vi "excel显示二维数组.vi"(8 "error in (no error)":errorcluster caption="错误输入（无错误）", 11 "数据二维":string[][](array[string])) -> (0 "error out":errorcluster caption="错误输出")   [LabVIEW 2014]
doc: "该模板用于创建子VI。"
panel:
  out "连接的字符串":string
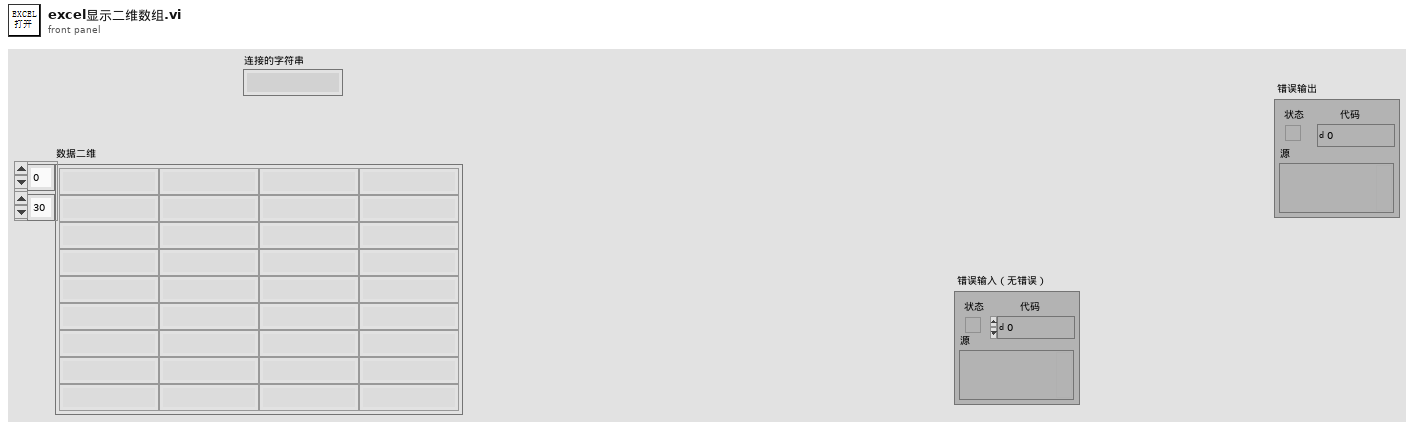
[diagram p1: front panel]
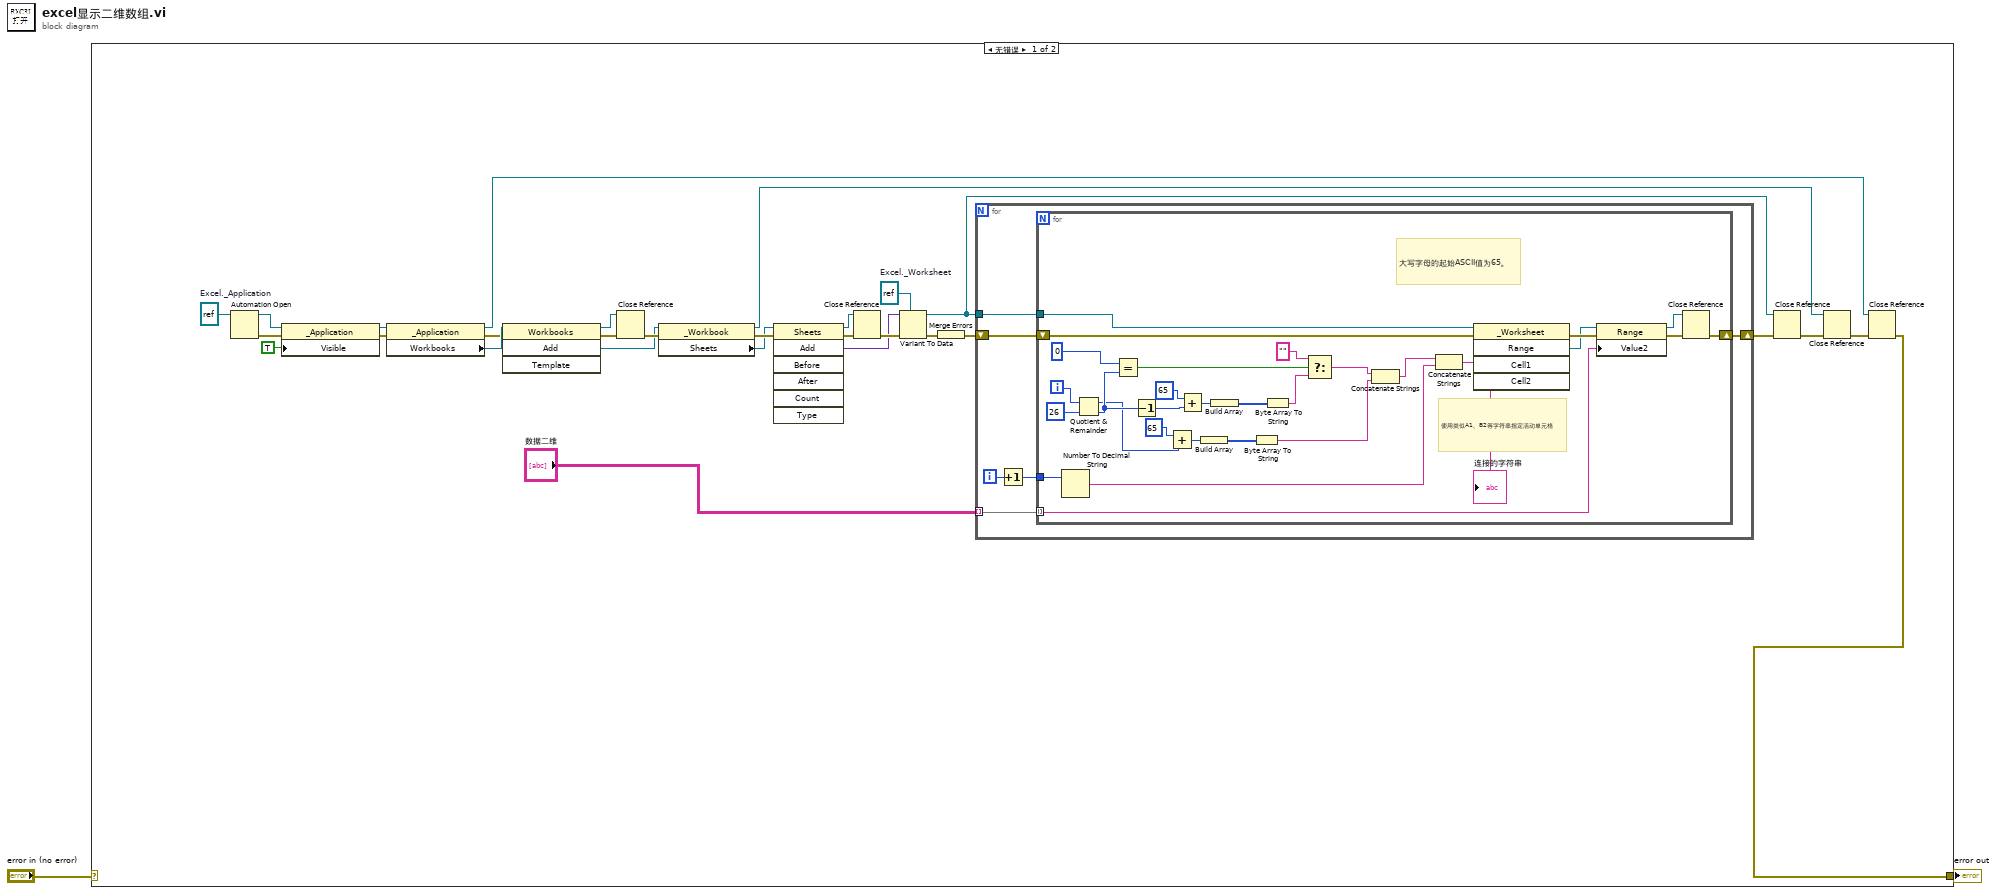
[diagram p0: block diagram]
diagram:
  n1 = case shown="无错误" "error in (no error)" {
    selector: "error in (no error)" -> [_ w67]
    tunnel: [w3 w67] -> w1
    frame No Error {
      w10 = refnum<k7> refnum  # Excel._Worksheet
      w26 = refnum<k7> refnum  # Excel._Application
      n2 = Automation Open(Automation Refnum=w26) -> (Automation Refnum=w27:refnum<k7>, error out=w28:errorcluster)  [unwired: 1 in, 2 out]
      n3 = property class="_Application"(reference=w27, error in=w28, "Visible"=TRUE) -> (reference out=w19:refnum<k7>, error out=w21:errorcluster)
      n4 = property class="_Application"(reference=w19, error in=w21) -> (reference out=w16:refnum<k7>, error out=w24:errorcluster, "Workbooks"=w25:refnum<k7>)
      n5 = invoke class="Workbooks" method="Add"(reference=w25, error in=w24) -> (reference out=w22:refnum<k7>, error out=w23:errorcluster, "Add"=w17:refnum<k7>)  [unwired: 2 in, 1 out]
      n6 = Close Reference(reference=w22, error in (no error)=w23) -> (error out=w18:errorcluster)
      n7 = property class="_Workbook"(reference=w17, error in=w18) -> (reference out=w14:refnum<k7>, error out=w8:errorcluster, "Sheets"=w7:refnum<k7>)
      n8 = invoke class="Sheets" method="Add"(reference=w7, error in=w8) -> (reference out=w11:refnum<k7>, error out=w12:errorcluster, "Add"=w9:variant)  [unwired: 5 in, 4 out]
      n9 = Close Reference(reference=w11, error in (no error)=w12) -> (error out=w13:errorcluster)
      n10 = Variant To Data(error in=w13, type=w10, Variant=w9) -> (data=w15:refnum<k7>, error out=w6:errorcluster)
      n11 = Merge Errors(w6) -> (w5:errorcluster)
      n12 = for {
        shift-right: [w36] -> w29
        shift-left: w5 -> [w37]
        tunnel: w15 -> [w35]
        tunnel: "数据二维" -> [w32] mode=indexing
        i -> [w34]
        n13 = Increment(x=w34) -> (x+1=w33:i32)
        n14 = for {
          shift-right: [w62] -> w36
          shift-left: w37 -> [w60]
          tunnel: w35 -> [w59]
          tunnel: w33 -> [w56]
          tunnel: w32 -> [w64] mode=indexing
          i -> [w53]
          # "使用类似A1、B2等字符串指定活动单元格"
          # "大写字母的起始ASCII值为65。"
          n15 = Number To Decimal String(number=w56) -> (decimal integer string=w55:string)  [unwired: 1 in]
          n16 = Quotient & Remainder(x=w53, y=26) -> (x-y*floor(x/y)=w39:i32, floor(x/y)=w40:i32)
          n17 = Equal?(x=0, y=w40) -> (x = y?=w46:bool)
          n18 = Decrement(x=w40) -> (x-1=w47:i32)
          n19 = Add(x=65, y=w39) -> (x+y=w57:i32)
          n20 = Add(x=65, y=w47) -> (x+y=w49:i32)
          n21 = Build Array(w57) -> (w38:i32[])
          n22 = Build Array(w49) -> (w50:i32[])
          n23 = Byte Array To String(unsigned byte array=w38) -> (string=w42:string)
          n24 = Byte Array To String(unsigned byte array=w50) -> (string=w44:string)
          n25 = Select(t="" ("十进制整型字符串"), s=w46, f=w44) -> (s? t:f=w43:string)
          n26 = Concatenate Strings(w43, w42) -> (w41:string)
          n27 = Concatenate Strings(w41, w55) -> (w54:string)
          "连接的字符串" <- w54
          n28 = invoke class="_Worksheet" method="Range"(reference=w59, error in=w60, "Cell1"=w54) -> (error out=w66:errorcluster, "Range"=w65:refnum<k7>)  [unwired: 2 in, 3 out]
          n29 = property class="Range"(reference=w65, error in=w66, "Value2"=w64) -> (reference out=w61:refnum<k7>, error out=w63:errorcluster)
          n30 = Close Reference(reference=w61, error in (no error)=w63) -> (error out=w62:errorcluster)
        }
      }
      n31 = Close Reference(reference=w15, error in (no error)=w29) -> (error out=w31:errorcluster)
      n32 = Close Reference(reference=w14, error in (no error)=w31) -> (error out=w30:errorcluster)
      n33 = Close Reference(reference=w16, error in (no error)=w30) -> (error out=w3:errorcluster)
    }
    frame Error {
    }
  }
  "error out" <- w1
